vi "Get Node Attributes.vi"(8 "error in (no error)":errorcluster, 11 "node in":refnum<k20>) -> (0 "error out":errorcluster, 1 "uid":string, 2 "class":string, 3 "node out":refnum<k20>, 4 "Array?":bool, 5 "Value":string, 7 "Name":string)   [LabVIEW 2023, in "VILab.lvlib"]
uses:
  VILab.lvlib
  <vilib>/xml/Close Reference(Node).vi
  <resource>/objmgr/DOMUserDefRef.rc
  <vilib>/xml/NI_XML.lvlib
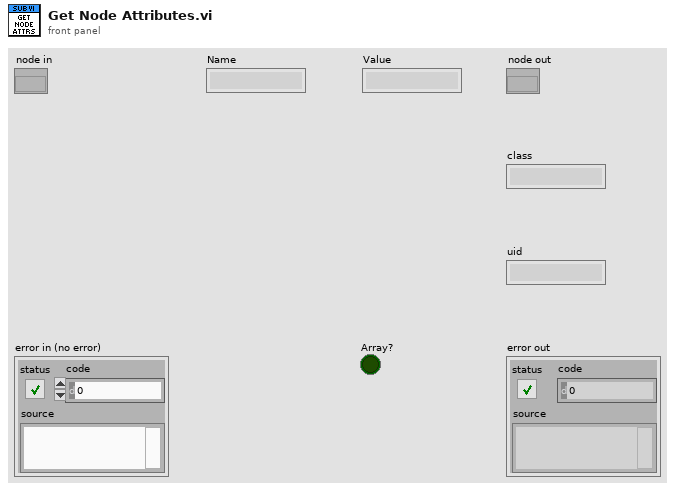
[diagram p1: front panel]
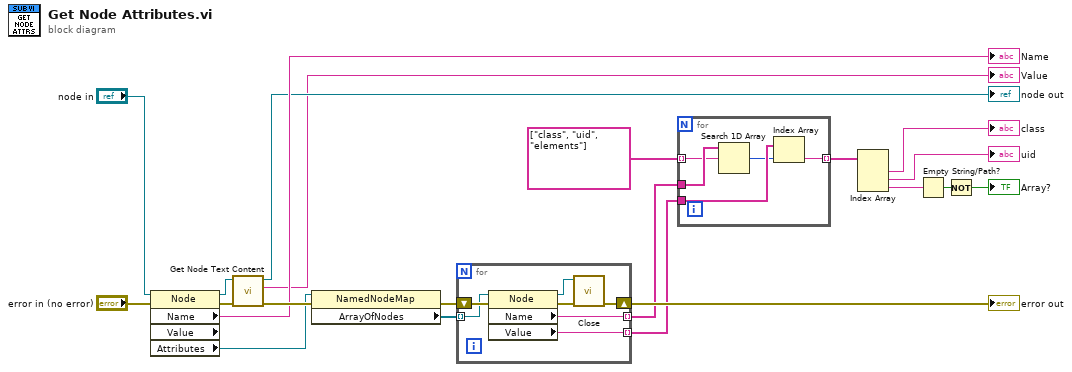
[diagram p0: block diagram]
diagram:
  n1 = property class="Node" props=["Name", "Value", "Attributes"](reference="node in", error in="error in (no error)") -> (reference out=w3:refnum<k20>, error out=w18:errorcluster, "Name"=→"Name":string, "Attributes"=w4:refnum<k20>)  [unwired: 1 out]
  n2 = call <vilib>:"Get Node Text Content.vi"("error in (no error)"=w18, "node in"=w3) -> ("error out"=w17:errorcluster, "node text"=→"Value":string, "node out"=→"node out":refnum<k20>)  [unwired: 7 in]
  n3 = property class="NamedNodeMap"(reference=w4, error in=w17) -> (error out=w21:errorcluster, "ArrayOfNodes"=w16:refnum<k20>[])  [unwired: 1 out]
  n4 = for {
    tunnel: w16 -> [w25] mode=indexing
    tunnel: [w24] -> w15 mode=indexing
    tunnel: [w23] -> w14 mode=indexing
    shift-right: [w26] -> w19
    shift-left: w21 -> [w28]
    n5 = property class="Node"(reference=w25, error in=w28) -> (reference out=w22:refnum<k20>, error out=w27:errorcluster, "Name"=w24:string, "Value"=w23:string)
    n6 = call-poly <vilib>:"Close.vi"("error in (no error)"=w27, "node"=w22) -> ("error out"=w26:errorcluster)  [unwired: 7 in]
  }
  "error out" <- w19
  n7 = for {
    tunnel: w15 -> [w33]
    tunnel: w14 -> [w31]
    tunnel: string[] ["class", "uid", "elements"] -> [w32] mode=indexing
    tunnel: [w29] -> w12 mode=indexing
    n8 = Search 1D Array(1D array=w33, element=w32) -> (index of element=w30:i32)  [unwired: 1 in]
    n9 = Index Array(array=w31, index=w30) -> (element=w29:string)
  }
  n10 = Index Array(array=w12) -> (element #1=→"class":string, element #2=→"uid":string, element #3=w8:string)  [unwired: 3 in]
  n11 = Empty String/Path?(string/path=w8) -> (empty?=w7:bool)
  n12 = Not(x=w7) -> (.not. x?=→"Array?":bool)
